vi "Push_Multi_Wrapping_More.vi"() -> ()   [LabVIEW 2024, in "POTCircularBuffer.Tests.Units.lvlib"]
uses:
  POTCircularBuffer.Tests.Units.lvlib
  <vilib>/addons/_JKI Toolkits/Caraya/classes/Assert/Assert.lvclass
  <vilib>/addons/_JKI Toolkits/Caraya/classes/Test/Test.lvclass
  POTTypedCircularBuffer.lvclass
  Type.ctl
  <vilib>/addons/_JKI Toolkits/Caraya/classes/Assert/Assert Equal Value and Type_Variant.vi
  <vilib>/addons/_JKI Toolkits/Caraya/classes/Assert/Assert Equal Value_Variant.vi
panel:
  out "remaining elements":T1[](array[typedef])
  out "Copied Buffer":T1[](array[typedef])
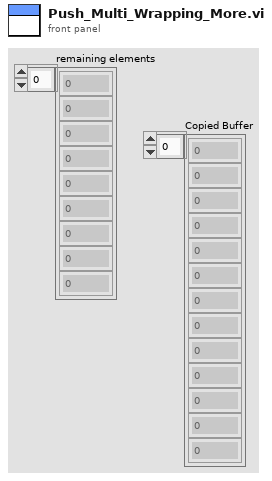
[diagram p1: front panel]
types:
  T1 = typedef "POTTypedCircularBuffer.lvclass/Type.ctl" = i32
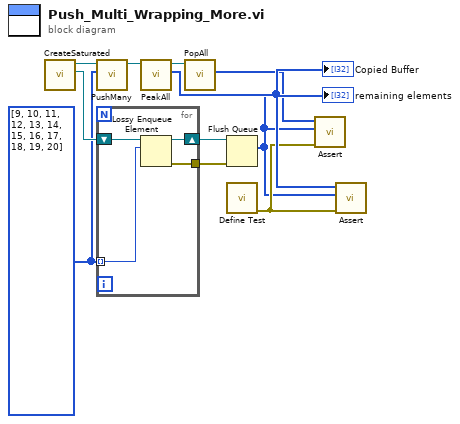
[diagram p0: block diagram]
diagram:
  w5 = T1[] [9, 10, 11, 12, 13, 14, 15, 16, 17, 18, 19, 20] ("Elements")
  n1 = call "CreateSaturated.vi"() -> ("Golden"=w8:refnum<queue>, "POTTypedCircularBuffer out"=w7:refnum<class "POTTypedCircularBuffer.lvclass">)  [unwired: 10 in]
  n2 = call "PushMany.vi"("Elements"=w5, "POTTypedCircularBuffer in"=w7) -> ("POTTypedCircularBuffer out"=w11:refnum<class "POTTypedCircularBuffer.lvclass">)  [unwired: 9 in]
  n3 = for {
    tunnel: [w15] -> w10
    shift-right: [w14] -> w9
    shift-left: w8 -> [w13]
    tunnel: w5 -> [w12] mode=indexing
    n4 = Lossy Enqueue Element(queue=w13, element=w12) -> (queue out=w14:refnum<queue>, error out=w15:errorcluster)  [unwired: 1 in, 2 out]
  }
  n5 = call "PeakAll.vi"("POTTypedCircularBuffer in"=w11) -> ("Copied Buffer"=w6:T1[], "POTTypedCircularBuffer out"=w2:refnum<class "POTTypedCircularBuffer.lvclass">)  [unwired: 9 in]
  "Copied Buffer" <- w6
  n6 = call "PopAll.vi"("POTTypedCircularBuffer in"=w2) -> ("Flushed Buffer"=w1:T1[])  [unwired: 9 in, 1 out]
  n7 = Flush Queue(queue=w9, error in (no error)=w10) -> (remaining elements=w3:T1[])  [unwired: 2 out]
  "remaining elements" <- w3
  n8 = call <vilib>:"Define Test.vi"() -> ("error out"=w4:errorcluster)  [unwired: 10 in, 1 out]
  n9 = call-poly <vilib>:"Assert.vi"("error in (no error)"=w4, "Y"=w3, "X"=w1) -> ()  [unwired: 7 in, 2 out]
  n10 = call-poly <vilib>:"Assert.vi"("error in (no error)"=w4, "Y"=w3, "X"=w6) -> ()  [unwired: 7 in, 2 out]
